vi "Find Insertion Point.vi"(7 "State":T1={"Prompt"="Click to add", "Listbox"=refnum, "Required"={"Strings"=[], "Bottom"=FALSE, "Italic"=FALSE, "FG"=0, "BG"=16777215, "Bold"=FALSE}, "Items"=[], "Req'd"=[], "Events"={"Items Changed"=refnum, "List Changed"=refnum}, "Max Rows"=-1, "Default name"=""}) -> (4 "Append":bool, 8 "Insert at":i32)   [LabVIEW 2020, in "KListboxEx.xctl"]
uses:
  KListboxEx.xctl
  State.ctl
  Required.ctl
  Events.ctl
  Event Action.ctl
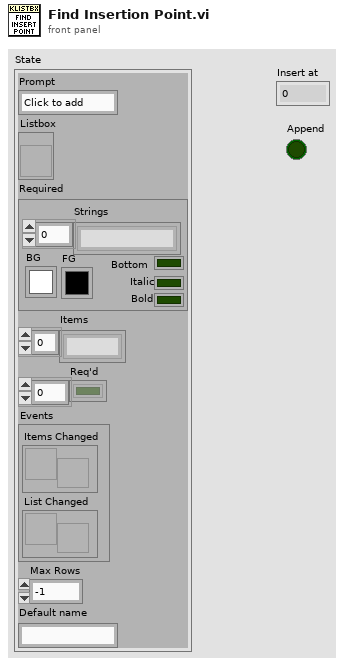
[diagram p1: front panel]
types:
  T1 = typedef "KListboxEx.xctl/State.ctl" = cluster{"Prompt":string, "Listbox":refnum<vi>, "Required":T2, "Items":string[], "Req'd":bool[], "Events":T3, "Max Rows":i32, "Default name":string}
  T2 = typedef "KListboxEx.xctl/Required.ctl" = cluster{"Strings":string[], "Bottom":bool, "Italic":bool, "FG":u32, "BG":u32, "Bold":bool}
  T3 = typedef "KListboxEx.xctl/Events.ctl" = cluster{"Items Changed":refnum<user-event>, "List Changed":refnum<user-event>}
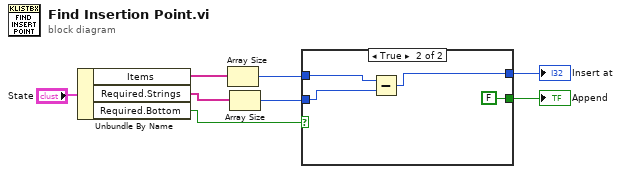
[diagram p0: block diagram]
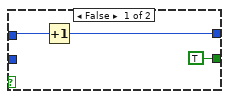
[diagram p2: hidden frame]
diagram:
  n1 = Unbundle By Name("State") -> ("Items"=w7:string[], "Required.Strings"=w6:string[], "Required.Bottom"=w5:bool)
  n2 = Array Size(array=w7) -> (size(s)=w3:i32)
  n3 = Array Size(array=w6) -> (size(s)=w4:i32)
  n4 = case shown="True" w5 {
    tunnel: w4 -> [_ w14]
    tunnel: w3 -> [w11 w15]
    tunnel: [w10 w13] -> w2
    tunnel: [TRUE FALSE] -> w1
    frame False {
      n5 = Increment(x=w11) -> (x+1=w10:i32)
    }
    frame True {
      n6 = Subtract(x=w15, y=w14) -> (x-y=w13:i32)
    }
  }
  "Insert at" <- w2
  "Append" <- w1
